vi "Untitled 1.vi"() -> ()   [LabVIEW 2021]
panel:
  out "BOOLEAN CONSTANT":bool
  out "STRING CONSTANT":string
  out "NUMERIC CONSTANT":i32
  in  "Boolean 2":bool
  in  "String":string
  in  "Numeric":dbl
  in  "Boolean":bool
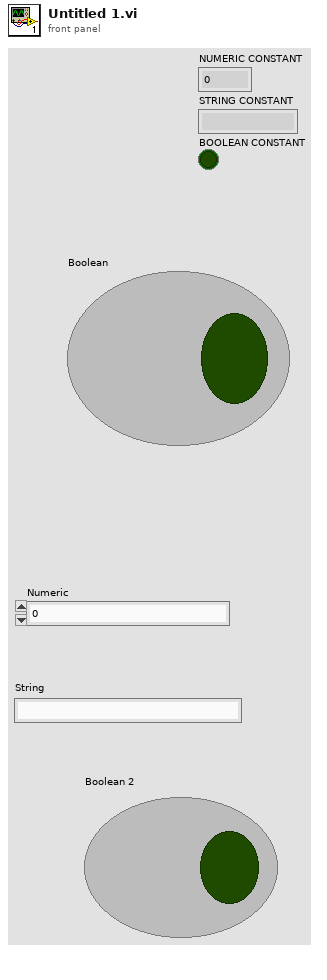
[diagram p1: front panel]
types:
  T1 = cluster{"NUMERIC CONSTANT":i32, "STRING CONSTANT":string, "BOOLEAN CONSTANT":bool}
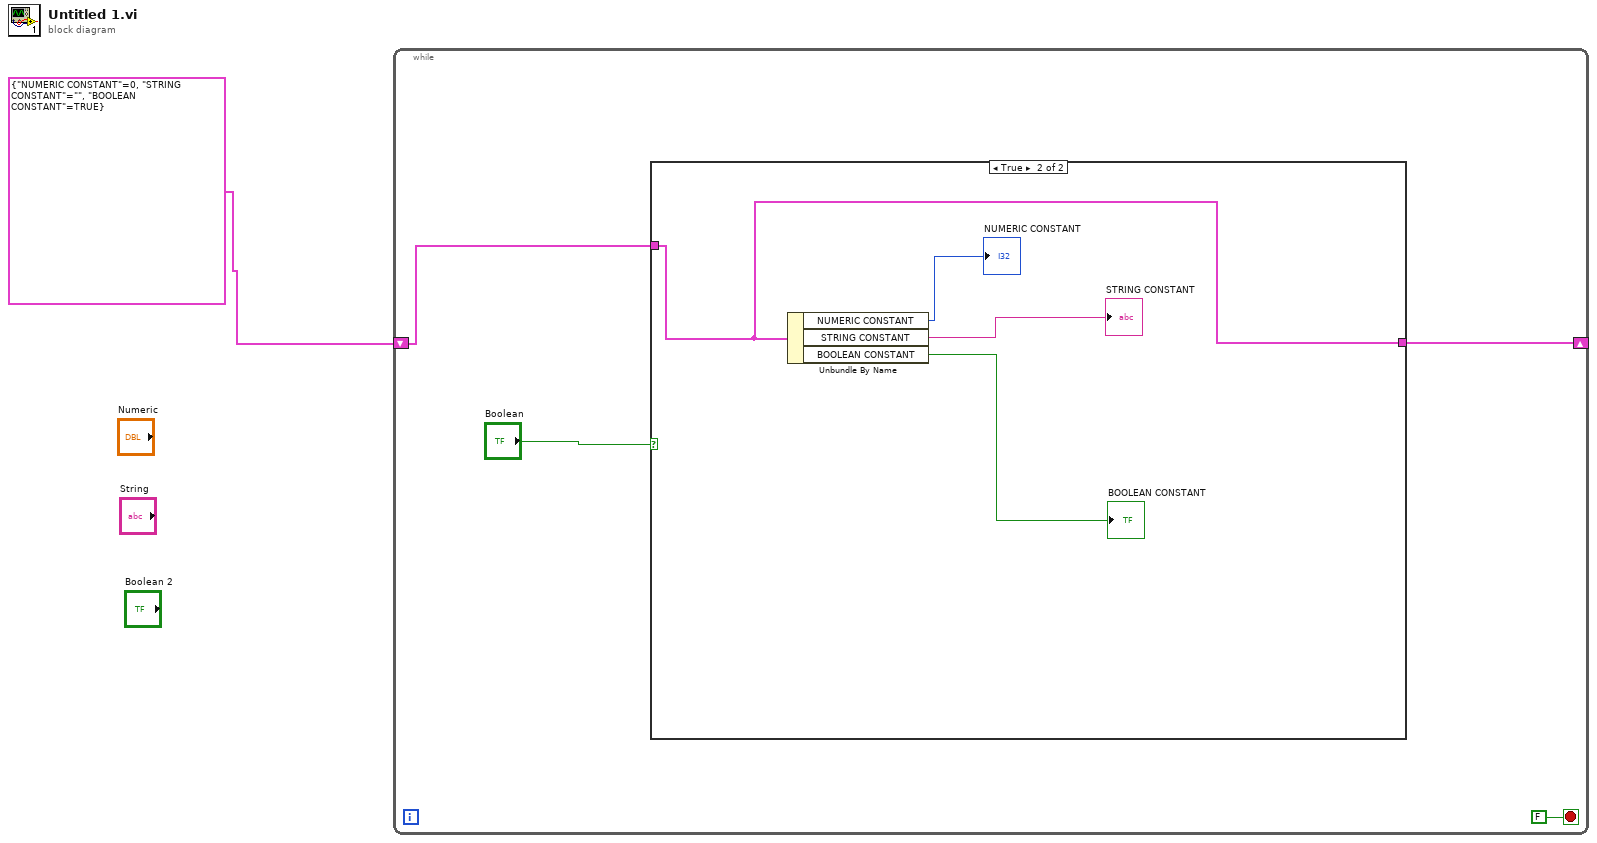
[diagram p0: block diagram]
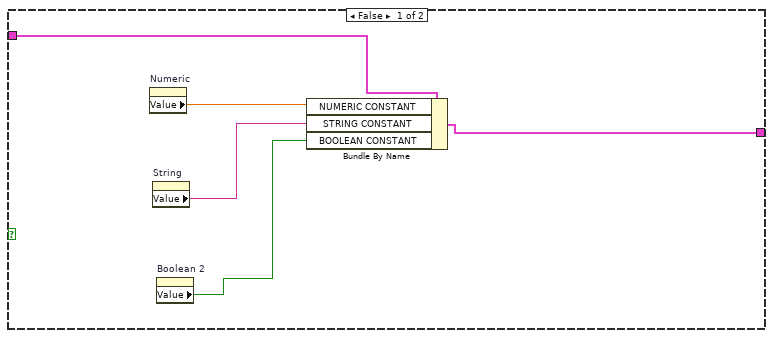
[diagram p2: hidden frame]
diagram:
  n1 = while {
    shift-right: [w4] -> _
    shift-left: T1 {"NUMERIC CONSTANT"=0, "STRING CONSTANT"="", "BOOLEAN CONSTANT"=TRUE} -> [w3]
    stop <- FALSE stop-if-true
    n2 = case shown="True" "Boolean" {
      tunnel: w3 -> [w10 w11]
      tunnel: [w6 w11] -> w4
      frame False {
        n3 = property on="Numeric" class="DigNum (strict)"() -> ("Value"=w9:dbl)  [unwired: 2 in, 2 out]
        n4 = property on="String" class="Str"() -> ("Value"=w8:string)  [unwired: 2 in, 2 out]
        n5 = property on="Boolean 2" class="Bool (strict)"() -> ("Value"=w7:bool)  [unwired: 2 in, 2 out]
        n6 = Bundle By Name(cluster=w10, "NUMERIC CONSTANT"=w9, "STRING CONSTANT"=w8, "BOOLEAN CONSTANT"=w7) -> (w6:T1)
      }
      frame True {
        n7 = Unbundle By Name(w11) -> ("NUMERIC CONSTANT"=→"NUMERIC CONSTANT":i32, "STRING CONSTANT"=→"STRING CONSTANT":string, "BOOLEAN CONSTANT"=→"BOOLEAN CONSTANT":bool)
      }
    }
  }
